vi "Latch with Reset.vi"(10 "reset":bool, 11 "signal":bool) -> (3 "latched signal":bool)   [LabVIEW 2013, in "I2S-TDM.lvlib"]
uses:
  I2S-TDM.lvlib
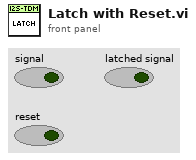
[diagram p1: front panel]
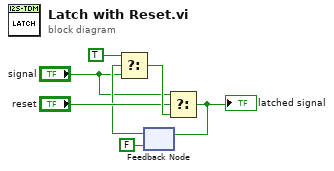
[diagram p0: block diagram]
diagram:
  n1 = feedback #1(FALSE ("rising edge?")) -> (w2:bool)
  n2 = Select(t=TRUE, s=w2, f="signal") -> (s? t:f=w4:bool)
  n3 = Select(t="signal", s="reset", f=w4) -> (s? t:f=w5:bool)
  "latched signal" <- w5
  n4 = feedback-in #1(w5) -> ()
